vi "mqttCmdBuildVarHdr.vi"(0 "_mqtt in":refnum<class "mqttCmdSubscribe.lvclass">, 11 "error in (no error)":errorcluster) -> (4 "_mqtt out":refnum<class "mqttCmdSubscribe.lvclass">, 8 "variableHeader":u8[](array[numeric]) format="%02x", 15 "error out":errorcluster)   [LabVIEW 2022 SP3, in "mqttCmdSubscribe.lvclass"]
uses:
  mqttCmdSubscribe.lvclass
  D:/Mac study folder/2022Fall/3CC3/_2022CCFinal/SRA_labview_ubidots/class/mqtt/mqttCmd/mqttCmd.lvclass
  mqttCmd.lvclass/mqttCmd.ctl
  mqttCmd.lvclass
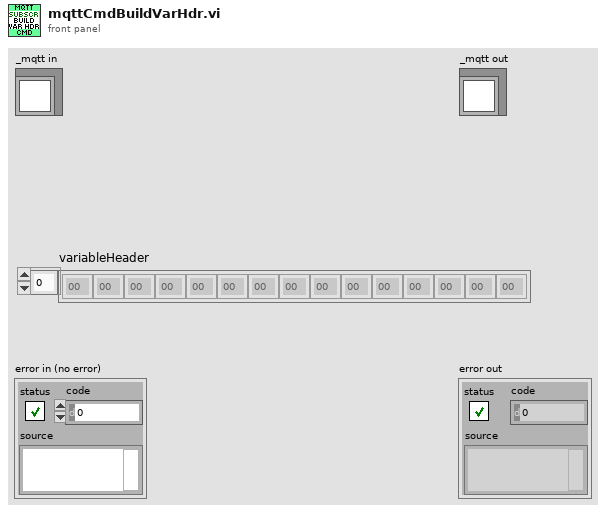
[diagram p1: front panel]
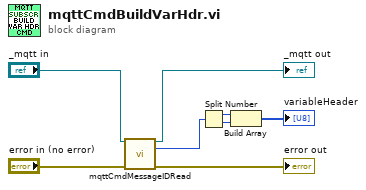
[diagram p0: block diagram]
diagram:
  n1 = call "mqttCmdMessageIDRead.vi"("mqttBrokerCommand in"="_mqtt in", "error in (no error)"="error in (no error)") -> ("mqttBrokerCommand out"=→"_mqtt out":refnum<class "mqttCmdSubscribe.lvclass">, "messageID"=w1:u16, "error out"=→"error out":errorcluster)  [unwired: 11 in]
  n2 = Split Number(x=w1) -> (hi(x)=w8:u8, lo(x)=w7:u8)
  n3 = Build Array(w8, w7) -> (→"variableHeader":u8[])
